vi "Initialize.vi"(8 "error in":errorcluster, 10 "shared resources":refnum<class "Shared Resources.lvclass">, 11 "Rx Execution Unit Implementation in":refnum<class "Rx Execution Unit.lvclass">) -> (0 "error out":errorcluster, 3 "Rx Execution Unit Implementation out":refnum<class "Rx Execution Unit.lvclass">)   [LabVIEW 2020, in "Ballard MIL-STD-1553 Engine.lvlib" / "Implementation.lvlib" / "Rx Execution Unit.lvclass"]
uses:
  Rx Execution Unit.lvclass
  C:/dev/niveristand-ballard-milStd1553-custom-device/Source/Custom Device Support/Engine/Implementation/Execution Unit/Execution Unit.lvclass
  Interfaces/Shared Resources/Shared Resources.lvclass
  Execution Unit/Execution Unit.lvclass/Execution Unit.ctl
  Rx Execution Unit.lvclass/Rx Execution Unit.ctl
  Execution Unit/Execution Unit.lvclass
  Custom Device/Custom Device.lvlib
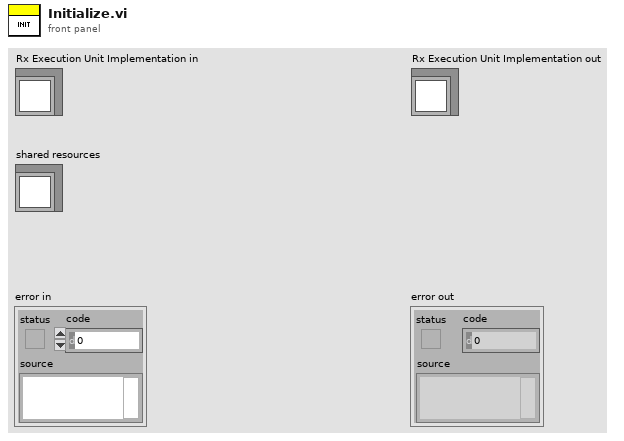
[diagram p1: front panel]
types:
  T1 = typedef "1553 Channel.ctl" = cluster{"HW channel":u16, "terminals":T2[], "messages":T4[], "acyclic frame names":string[]}
  T2 = typedef "Terminal Name and Address.ctl" = cluster{"name":string, "terminal address":T3}
  T3 = typedef "Address.ctl" = u16
  T4 = typedef "Message Definition.ctl" = cluster{"name":string, "message type":T5, "endpoint Rx":T6, "endpoint Tx":T6, "mode code":u16, "number of words":u16, "parameters":cluster{"name":string, "default value":dbl, "unit":string, "parameter definition":T7}[], "create timestamp channel":bool}
  T5 = typedef "Message Type.ctl" = string
  T6 = typedef "Terminal Endpoint.ctl" = cluster{"terminal address":T3, "subaddress":T3}
  T7 = typedef "Parameter Definition.ctl" = cluster{"start index":i32, "size (bits)":i32, "encoding":enum16{"BNR", "BCD", "Discrete"}, "signed":bool, "multiplier":dbl, "offset":dbl}
  T8 = typedef "Map of Messages to Value Indexes.ctl" = map{T9, i32}
  T9 = typedef "Message Map Key.ctl" = cluster{"HW channel":u16, "terminal address":u16, "subaddress":u16, "mode code":u16}
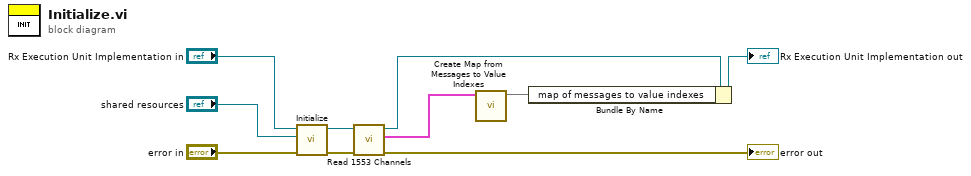
[diagram p0: block diagram]
diagram:
  n1 = call-parent "Initialize.vi"("error in"="error in", "shared resources"="shared resources", "Execution Unit Implementation in"="Rx Execution Unit Implementation in") -> ("error out"=w6:errorcluster, "Execution Unit Implementation out"=w7:refnum<class "Rx Execution Unit.lvclass">)  [unwired: 7 in]
  n2 = call "Read 1553 Channels.vi"("error in (no error)"=w6, "Execution Unit in"=w7) -> ("error out"=→"error out":errorcluster, "1553 channels"=w2:T1[], "Execution Unit out"=w4:refnum<class "Rx Execution Unit.lvclass">)  [unwired: 7 in]
  n3 = call "Create Map from Messages to Value Indexes.vi"("1553 channels"=w2) -> ("map from messages to value indexes"=w1:T8)  [unwired: 10 in]
  n4 = Bundle By Name(cluster=w4, "map of messages to value indexes"=w1) -> (→"Rx Execution Unit Implementation out":refnum<class "Rx Execution Unit.lvclass">)
